vi "Check.vi"(8 "error in (no error)":errorcluster, 11 "RPTID Data":cluster{"RPTID":u32, "VID":u32[]}[](array[cluster])) -> (0 "error out":errorcluster, 3 "S2F34":T1)   [LabVIEW 2020, in "SECS Scenarios.lvlib" / "33-RPTID Setup.lvclass"]
uses:
  33-RPTID Setup.lvclass
  SECS Communication/S2 Message Class/S2F34.ctl
  SECS Communication/SECS Data Class/Get RPTID Data.vi
  SECS Communication/SECS Data Class/Get SVID Data.vi
  SECS Communication/SECS Data Class/SECS Data Class.lvclass
  SECS Communication/S2 Message Class/S2 Message Class.lvclass
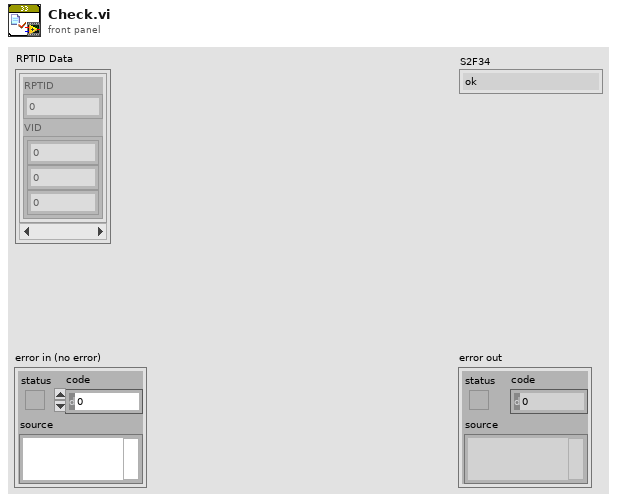
[diagram p1: front panel]
types:
  T1 = typedef "SECS Communication.lvlib/S2 Message Class.lvclass/S2F34.ctl" = enum16{"ok", "out of space", "invalid format", "1 or more RPTID already defined", "1 or more invalid VID"}
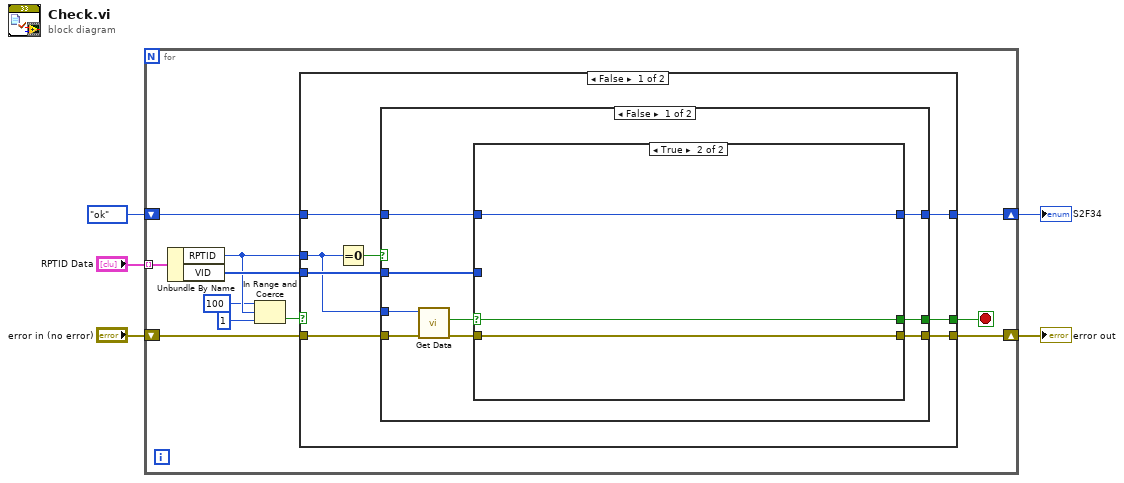
[diagram p0: block diagram]
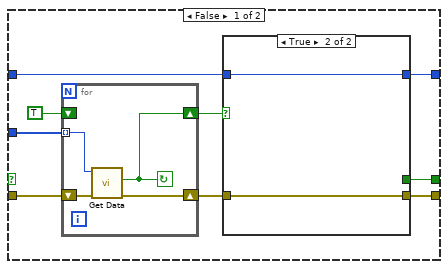
[diagram p2: hidden frame]
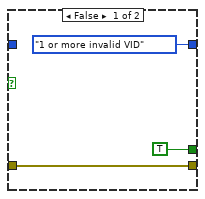
[diagram p3: hidden frame]
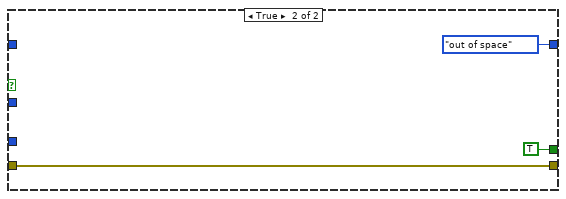
[diagram p4: hidden frame]
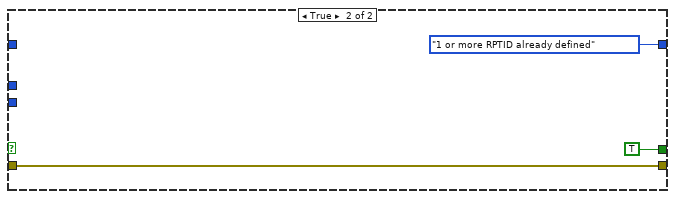
[diagram p5: hidden frame]
diagram:
  n1 = for {
    tunnel: "RPTID Data" -> [w16] mode=indexing
    shift-right: [w10] -> w2
    shift-left: "error in (no error)" -> [w15]
    shift-right: [w11] -> w1
    shift-left: S2F34."ok" ("S2F34") -> [w12]
    stop <- w13 stop-if-true
    n2 = Unbundle By Name(w16) -> ("RPTID"=w9:u32, "VID"=w14:u32[])
    n3 = In Range and Coerce(upper limit=u32 100, x=w9, lower limit=u32 1) -> (In Range?=w6:bool)  [unwired: 1 out]
    n4 = case shown="False" w6 {
      tunnel: w15 -> [w24 w60]
      tunnel: w14 -> [w23 _]
      tunnel: [w22 TRUE] -> w13
      tunnel: w12 -> [w21 _]
      tunnel: [w20 S2F34."1 or more RPTID already defined" ("S2F34")] -> w11
      tunnel: [w19 w60] -> w10
      tunnel: w9 -> [w18 _]
      frame False {
        n5 = Equal To 0?(x=w18) -> (x = 0?=w17:bool)
        n6 = case shown="False" w17 {
          tunnel: w24 -> [w33 w57]
          tunnel: w23 -> [w30 _]
          tunnel: [w29 TRUE] -> w22
          tunnel: w21 -> [w28 _]
          tunnel: [w27 S2F34."out of space" ("S2F34")] -> w20
          tunnel: [w26 w57] -> w19
          tunnel: w18 -> [w25 _]
          frame False {
            n7 = call-poly "Get Data.vi"("error in"=w33, "RPTID"=w25) -> ("error out"=w32:errorcluster, "Find?"=w31:bool)  [unwired: 7 in, 1 out]
            n8 = case shown="True" w31 {
              selector: w31 -> [_ w53]
              tunnel: w32 -> [w42 w54]
              tunnel: w30 -> [w36 _]
              tunnel: [w37 w53] -> w29
              tunnel: [w38 w54] -> w26
              tunnel: w28 -> [w40 w52]
              tunnel: [w39 w52] -> w27
              frame False {
                n9 = for {
                  shift-right: [w49] -> w41
                  shift-left: w42 -> [w51]
                  tunnel: w36 -> [w50] mode=indexing
                  shift-right: [w48] -> w34
                  shift-left: TRUE -> [_]
                  stop <- w48 continue-if-true
                  n10 = call-poly "Get Data.vi"("error in"=w51, "SVID"=w50) -> ("error out"=w49:errorcluster, "Find?"=w48:bool)  [unwired: 7 in, 1 out]
                }
                n11 = case shown="True" w34 {
                  tunnel: w41 -> [w44 w46]
                  tunnel: w40 -> [_ w47]
                  tunnel: [S2F34."1 or more invalid VID" ("S2F34") w47] -> w39
                  tunnel: [w44 w46] -> w38
                  tunnel: [TRUE _] -> w37
                  frame False {
                  }
                  frame True {
                  }
                }
              }
              frame True {
              }
            }
          }
          frame True {
          }
        }
      }
      frame True {
      }
    }
  }
  "error out" <- w2
  "S2F34" <- w1
